vi "Send instructions.vi"(8 "error in (no error)":errorcluster, 10 "instructions":string[](array[string]), 11 "Motor in":refnum<class "Motor.lvclass">) -> (0 "error out":errorcluster, 1 "error":bool, 2 "replies":string[](array[string]), 3 "Motor out":refnum<class "Motor.lvclass">, 4 "ok":bool)   [LabVIEW 2018, in "Motor.lvclass"]
uses:
  Motor.lvclass
  Motor.lvclass/Motor.ctl
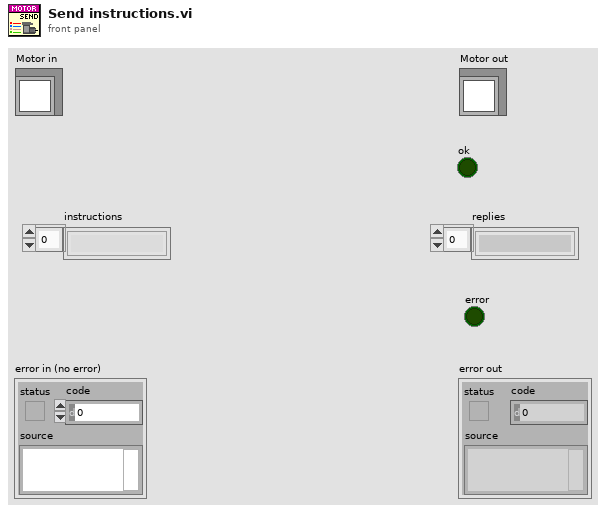
[diagram p1: front panel]
types:
  T1 = enum16{"Standard", "Buffered", "CRLF", "Immediate"}
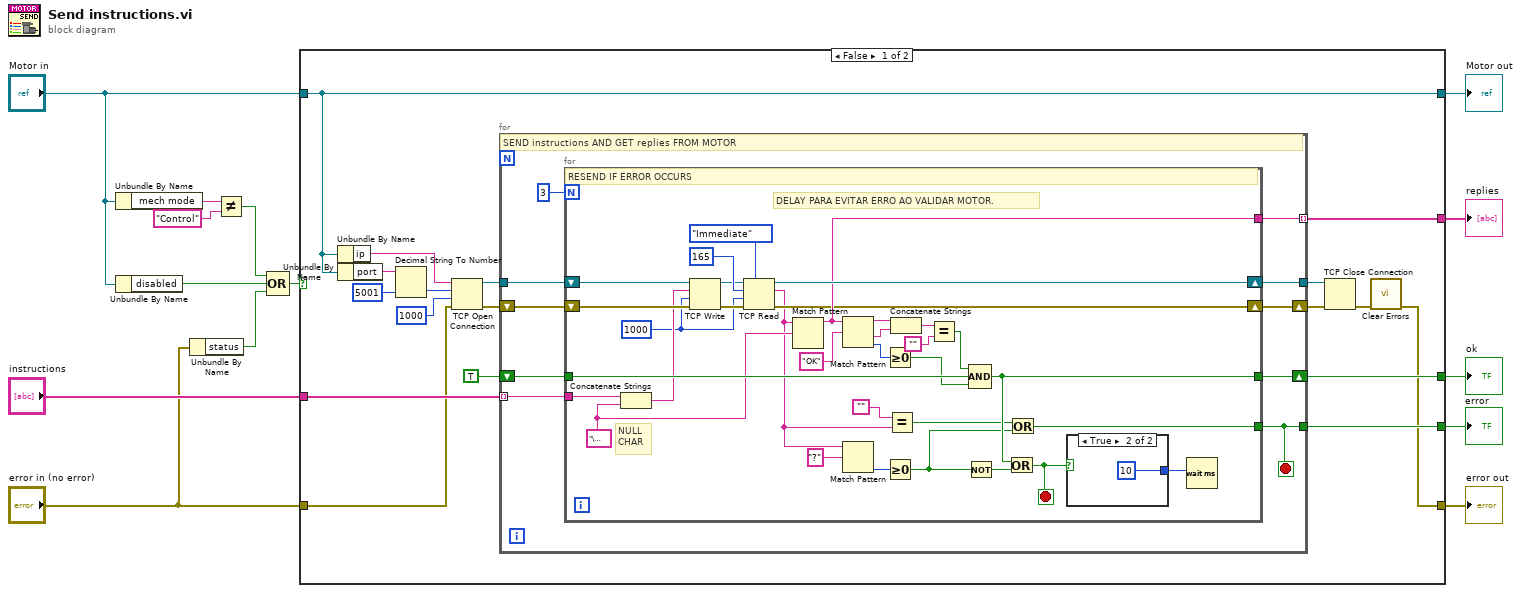
[diagram p0: block diagram]
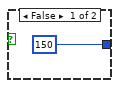
[diagram p2: hidden frame]
diagram:
  n1 = Unbundle By Name("Motor in") -> ("mech mode"=w7:string)
  n2 = Unbundle By Name("Motor in") -> ("disabled"=w4:bool)
  n3 = Unbundle By Name("error in (no error)") -> ("status"=w5:bool)
  n4 = Not Equal?(x=w7, y="Control") -> (x != y?=w1:bool)
  n5 = Compound Arithmetic op=OR(w1, w4, w5) -> (w3:bool)
  n6 = case shown="False" w3 {
    tunnel: [w16 w78] -> w14
    tunnel: [w32 w79] -> w13
    tunnel: "Motor in" -> [w32 w79]
    tunnel: "instructions" -> [w26 _]
    tunnel: [w23 _] -> w11
    tunnel: [w19 _] -> w10
    tunnel: [w18 _] -> w9
    tunnel: "error in (no error)" -> [w15 w78]
    frame False {
      n7 = Unbundle By Name(w32) -> ("ip"=w27:string)
      n8 = Unbundle By Name(w32) -> ("port"=w30:string)
      n9 = Decimal String To Number(string=w30, default (0L)=u16 5001 ("default (0 I32)")) -> (number=w28:u16)  [unwired: 1 in, 1 out]
      n10 = TCP Open Connection(address=w27, remote port or service name=w28, timeout ms (60000)=1000, error in (no error)=w15) -> (connection ID=w24:refnum<k5>, error out=w25:errorcluster)  [unwired: 1 in]
      n11 = for {
        tunnel: w26 -> [w42] mode=indexing
        tunnel: w24 -> [w40]
        tunnel: [w35] -> w23
        shift-right: [w39] -> w19
        shift-left: TRUE -> [w34]
        tunnel: [w38] -> w21
        shift-right: [w36] -> w20
        shift-left: w25 -> [w41]
        tunnel: [w37] -> w18 mode=indexing
        stop <- w35 stop-if-true
        # "SEND instructions AND GET replies FROM MOTOR"
        n12 = for {
          N: 3 -> [_]
          tunnel: w42 -> [w75]
          tunnel: [w71] -> w37
          tunnel: [w49] -> w35
          shift-right: [w70] -> w36
          shift-left: w41 -> [w74]
          shift-right: [w72] -> w38
          shift-left: w40 -> [w73]
          tunnel: w34 -> [w69]
          tunnel: [w51] -> w39
          stop <- w45 stop-if-true
          w63 = 1000 ("timeout ms (60000)")
          w55 = "\u0000" ("search string")
          # "DELAY PARA EVITAR ERRO AO VALIDAR MOTOR."
          # "NULL\nCHAR"
          # "RESEND IF ERROR OCCURS"
          n13 = Concatenate Strings(w75, w55) -> (w64:string)
          n14 = TCP Write(connection ID=w73, data in=w64, error in (no error)=w74, 9:w63) -> (connection ID out=w66:refnum<k5>, error out=w68:errorcluster)  [unwired: 1 out]
          n15 = TCP Read(connection ID=w66, bytes to read=165, error in (no error)=w68, 7:T1."Immediate" ("mode (standard)"), 9:w63) -> (connection ID out=w72:refnum<k5>, data out=w47:string, error out=w70:errorcluster)
          n16 = Match Pattern(string=w47, regular expression=w55) -> (before substring=w71:string)  [unwired: 1 in, 3 out]
          n17 = Match Pattern(string=w71, regular expression="OK" ("y")) -> (before substring=w57:string, after substring=w60:string, offset past match=w54:i32)  [unwired: 1 in, 1 out]
          n18 = Match Pattern(string=w47, regular expression="?") -> (offset past match=w62:i32)  [unwired: 1 in, 3 out]
          n19 = Greater Or Equal To 0?(x=w54) -> (x >= 0?=w52:bool)
          n20 = Greater Or Equal To 0?(x=w62) -> (x >= 0?=w50:bool)
          n21 = Equal?(x="", y=w47) -> (x = y?=w48:bool)
          n22 = Concatenate Strings(w57, w60) -> (w58:string)
          n23 = Equal?(x=w58, y="") -> (x = y?=w53:bool)
          n24 = Not(x=w50) -> (.not. x?=w44:bool)
          n25 = Compound Arithmetic op=AND(w53, w69, w52) -> (w51:bool)
          n26 = Or(x=w51, y=w44) -> (x .or. y?=w45:bool)
          n27 = Or(x=w48, y=w50) -> (x .or. y?=w49:bool)
          n28 = case shown="True" w45 {
            tunnel: [u32 150 ("milliseconds to wait") u32 10 ("milliseconds to wait")] -> w43
            frame False {
            }
            frame True {
            }
          }
          n29 = Wait (ms)(milliseconds to wait=w43) -> ()  [unwired: 1 out]
        }
      }
      n30 = TCP Close Connection(connection ID=w21, error in (no error)=w20) -> (error out=w17:errorcluster)  [unwired: 1 in, 1 out]
      n31 = call <vilib>:"Clear Errors.vi"("error in (no error)"=w17) -> ("error out"=w16:errorcluster)  [unwired: 5 in, 1 out]
    }
    frame True {
    }
  }
  "error out" <- w14
  "Motor out" <- w13
  "error" <- w11
  "ok" <- w10
  "replies" <- w9
